vi "logScanLog.vi"(8 "error in (no error)":errorcluster, 10 "File Name":string, 11 "Model in":refnum<class "Model.lvclass">) -> (0 "error out":errorcluster, 3 "Model out":refnum<class "Model.lvclass">)   [LabVIEW 2015, in "Model.lvclass"]
uses:
  Model.lvclass
  Typedefs/WriteDataFileInput.ctl
  Typedefs/WriteLogMessageInput.ctl
  Model.lvclass/Model.ctl
  TestLog/ITestLog/ITestLog.lvclass
  Typedefs/FAMTTypedefs.lvlib
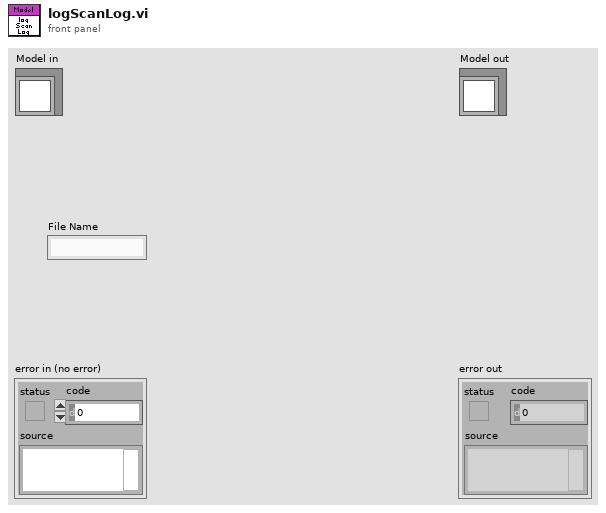
[diagram p1: front panel]
types:
  T1 = typedef "FAMTTypedefs.lvlib/WriteLogMessageInput.ctl" = cluster{"Description":string, "Data File":string}
  T2 = typedef "FAMTTypedefs.lvlib/WriteDataFileInput.ctl" = cluster{"File Name":string, "Output":string[]}
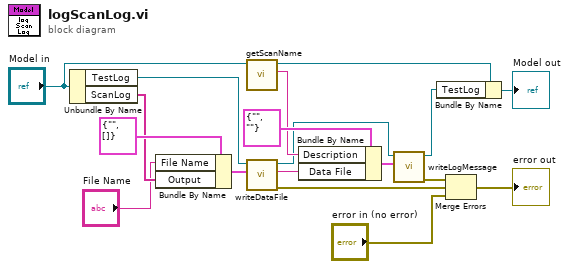
[diagram p0: block diagram]
diagram:
  n1 = Unbundle By Name("Model in") -> ("TestLog"=w18:refnum<class "ITestLog.lvclass">, "ScanLog"=w11:string[])
  n2 = Bundle By Name(cluster=T2 {"File Name"="", "Output"=[]} ("WriteDataFileInput"), "File Name"="File Name", "Output"=w11) -> (w12:T2)
  n3 = call "getScanName.vi"("Model in"="Model in") -> ("Scan Name"=w6:string, "Model out"=w4:refnum<class "Model.lvclass">)  [unwired: 8 in, 1 out]
  n4 = call-dynamic "writeDataFile.vi"("WriteDataFileInput"=w12, "ITestLog in"=w18) -> ("error out"=w16:errorcluster, "Relative Path"=w7:string, "ITestLog out"=w3:refnum<class "ITestLog.lvclass">)  [unwired: 7 in]
  n5 = Bundle By Name(cluster=T1 {"Description"="", "Data File"=""} ("WriteLogMessageInput"), "Description"=w6, "Data File"=w7) -> (w8:T1)
  n6 = call-dynamic "writeLogMessage.vi"("WriteLogMessageInput"=w8, "ITestLog in"=w3) -> ("error out"=w1:errorcluster, "ITestLog out"=w2:refnum<class "ITestLog.lvclass">)  [unwired: 8 in]
  n7 = Bundle By Name(cluster=w4, "TestLog"=w2) -> (→"Model out":refnum<class "Model.lvclass">)
  n8 = Merge Errors(w1, w16, "error in (no error)") -> (→"error out":errorcluster)
